vi "Reset Message Queue.vi"(8 "error in (no error)":errorcluster, 11 "Message Queue In":refnum<queue>) -> (0 "error out":errorcluster, 3 "Message Queue Out":refnum<queue>)   [LabVIEW 2023, in "HAF.lvlib"]
doc: "Empties the queue of any existing messages and adds an initialise message. This will create a known, good start point for processing."
uses:
  HAF.lvlib
  All Internal Message Ids.ctl
  Message.ctl
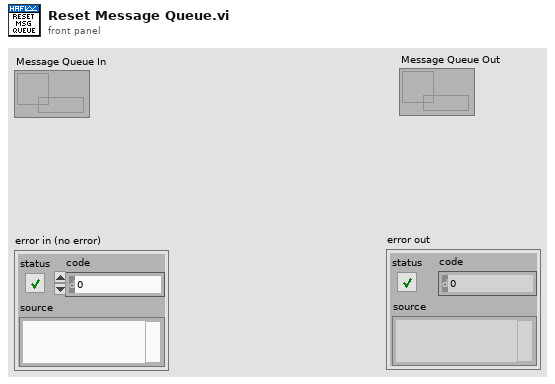
[diagram p1: front panel]
types:
  T1 = typedef "HAF.lvlib/All Internal Message Ids.ctl" = cluster{"Initialise":string, "Process":string, "Continue":string, "Done":string, "Pause":string, "Resume":string, "Stop":string, "Exit":string}
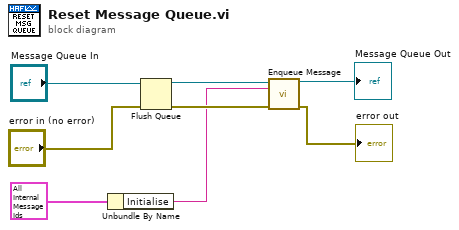
[diagram p0: block diagram]
diagram:
  n1 = Unbundle By Name(T1 {"Initialise"="Initialise", "Process"="Process", "Continue"="Continue", "Done"="Done", "Pause"="Pause", "Resume"="Resume", "Stop"="Stop", "Exit"="Exit"} ("Message Ids")) -> ("Initialise"=w3:string)
  n2 = Flush Queue(queue="Message Queue In", error in (no error)="error in (no error)") -> (queue out=w6:refnum<queue>, error out=w5:errorcluster)  [unwired: 1 out]
  n3 = call "Enqueue Message.vi"("Message Queue In"=w6, "Message Id"=w3, "error in (no error)"=w5) -> ("Message Queue Out"=→"Message Queue Out":refnum<queue>, "error out"=→"error out":errorcluster)  [unwired: 11 in]
